vi "lab1.vi"() -> ()   [LabVIEW 2011]
panel:
  out "Boolean 2":bool
  in  "Boolean":bool
  in  "Slide 2":dbl(slide) scale=0.0..10.0
  out "Meter":dbl(knob) scale=0.0..10.0
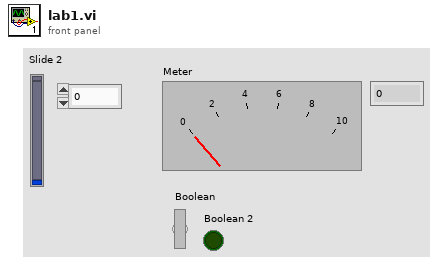
[diagram p1: front panel]
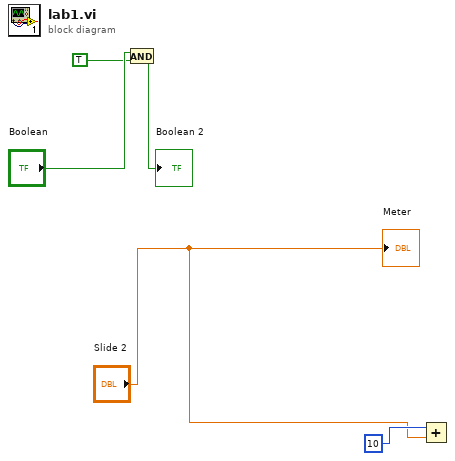
[diagram p0: block diagram]
diagram:
  n1 = And(x="Boolean", y=TRUE) -> (x .and. y?=→"Boolean 2":bool)
  n2 = Add(x=10, y="Slide 2") -> ()  [unwired: 1 out]
  "Meter" <- "Slide 2"
